vi "Fpga-Zero-out-Tkeep-bytes.vi"(10 "tkeep (MAC)":u8 format="%.0x", 11 "data_in":u32 format="%.0x") -> (3 "data_out":u32 format="%.0x")   [LabVIEW 2018]
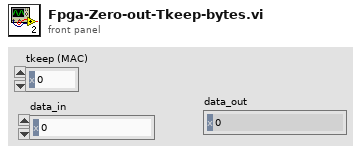
[diagram p1: front panel]
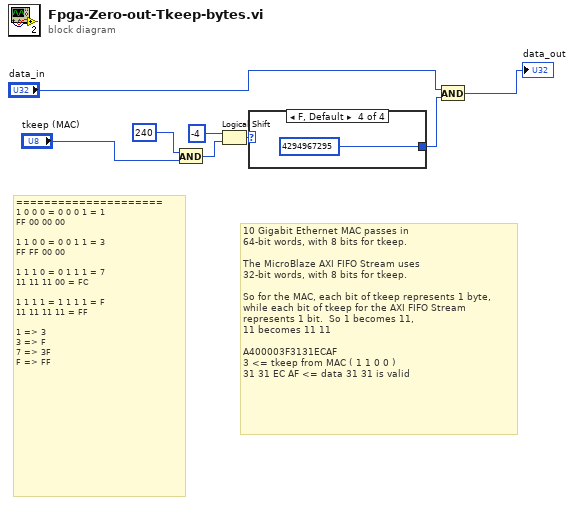
[diagram p0: block diagram]
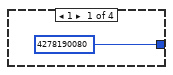
[diagram p2: hidden frame]
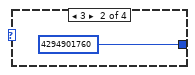
[diagram p3: hidden frame]
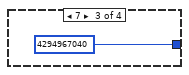
[diagram p4: hidden frame]
diagram:
  # "10 Gigabit Ethernet MAC passes in\n64-bit words, with 8 bits for tkeep.\n\nThe MicroBlaze AXI FIFO Stream uses\n32-bit words, with 8 bits for tkeep.\n\nSo for the MAC, each bit of tkeep represents 1 byte, \nwhile each bit of tkeep for the AXI FIFO Stream\nrepresents 1 bit.  So 1 becomes 11,\n11 becomes 11 11\n\nA400003F3131ECAF\n3 <= tkeep from MAC ( 1 1 0 0 )\n31 31 EC AF <= data 31 31 is valid"
  # "=====================\n1 0 0 0 = 0 0 0 1 = 1\nFF 00 00 00\n\n1 1 0 0 = 0 0 1 1 = 3\nFF FF 00 00\n\n1 1 1 0 = 0 1 1 1 = 7\n11 11 11 00 = FC\n\n1 1 1 1 = 1 1 1 1 = F\n11 11 11 11 = FF\n\n1 => 3\n3 => F\n7 => 3F\nF => FF"
  n1 = And(x=u8 240, y="tkeep (MAC)") -> (x .and. y?=w4:u8)
  n2 = Logical Shift(y=i16 -4, x=w4) -> (x << y=w7:u8)
  n3 = case shown="F, Default" w7 {
    tunnel: [u32 4278190080 ("y") u32 4294901760 ("y") u32 4294967040 ("y") u32 4294967295 ("y")] -> w3
    frame 1 {
    }
    frame 3 {
    }
    frame 7 {
    }
    frame 15, Default {
    }
  }
  n4 = And(x="data_in", y=w3) -> (x .and. y?=→"data_out":u32)
